vi "Word_Write_Text.vi"(8 "error in (no error)":errorcluster, 9 "text (\"\")":string, 10 "bookmark (\"\")":string="A_Faz_Frekans_3_3", 11 "report in":refnum<class "NI_report.lvclass">) -> (0 "error out":errorcluster, 3 "report out":refnum<class "NI_report.lvclass">)   [LabVIEW 2014]
doc: "This VI demonstrates the use of ActiveX to write a table into a Microsoft Excel worksheet."
uses:
  <vilib>/Utility/NIReport.llb/NI_report.lvclass
  <vilib>/Utility/NIReport.llb/Word/NI_Word.lvclass
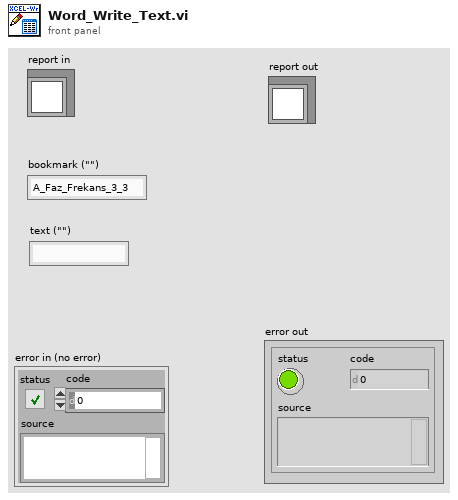
[diagram p1: front panel]
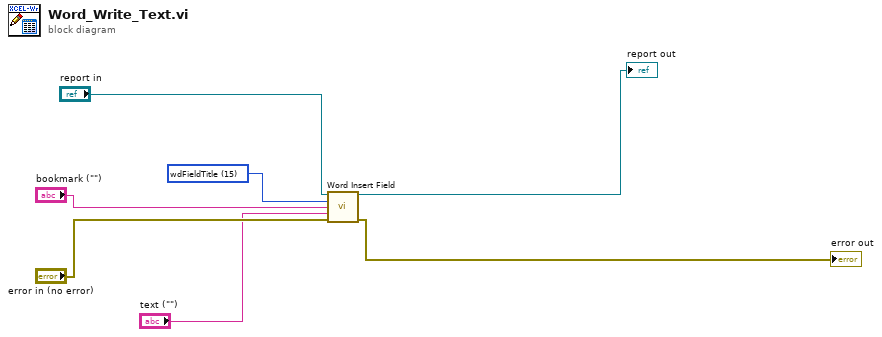
[diagram p0: block diagram]
diagram:
  w3 = 15 items=["wdFieldEmpty"=-1, "wdFieldRef"=3, "wdFieldIndexEntry"=4, "wdFieldFootnoteRef"=5, "wdFieldSet"=6, "wdFieldIf"=7, "wdFieldIndex"=8, "wdFieldTOCEntry"=9, "wdFieldStyleRef"=10, "wdFieldRefDoc"=11, "wdFieldSequence"=12, "wdFieldTOC"=13, "wdFieldInfo"=14, "wdFieldTitle"=15, "wdFieldSubject"=16, "wdFieldAuthor"=17, "wdFieldKeyWord"=18, "wdFieldComments"=19, "wdFieldLastSavedBy"=20, "wdFieldCreateDate"=21, "wdFieldSaveDate"=22, "wdFieldPrintDate"=23, "wdFieldRevisionNum"=24, "wdFieldEditTime"=25, "wdFieldNumPages"=26, "wdFieldNumWords"=27, "wdFieldNumChars"=28, "wdFieldFileName"=29, "wdFieldTemplate"=30, "wdFieldDate"=31, "wdFieldTime"=32, "wdFieldPage"=33, "wdFieldExpression"=34, "wdFieldQuote"=35, "wdFieldInclude"=36, "wdFieldPageRef"=37, "wdFieldAsk"=38, "wdFieldFillIn"=39, "wdFieldData"=40, "wdFieldNext"=41, "wdFieldNextIf"=42, "wdFieldSkipIf"=43, "wdFieldMergeRec"=44, "wdFieldDDE"=45, "wdFieldDDEAuto"=46, "wdFieldGlossary"=47, "wdFieldPrint"=48, "wdFieldFormula"=49, "wdFieldGoToButton"=50, "wdFieldMacroButton"=51, "wdFieldAutoNumOutline"=52, "wdFieldAutoNumLegal"=53, "wdFieldAutoNum"=54, "wdFieldImport"=55, "wdFieldLink"=56, "wdFieldSymbol"=57, "wdFieldEmbed"=58, "wdFieldMergeField"=59, "wdFieldUserName"=60, "wdFieldUserInitials"=61, "wdFieldUserAddress"=62, "wdFieldBarCode"=63, "wdFieldDocVariable"=64, "wdFieldSection"=65, "wdFieldSectionPages"=66, "wdFieldIncludePicture"=67, "wdFieldIncludeText"=68, "wdFieldFileSize"=69, "wdFieldFormTextInput"=70, "wdFieldFormCheckBox"=71, "wdFieldNoteRef"=72, "wdFieldTOA"=73, "wdFieldTOAEntry"=74, "wdFieldMergeSeq"=75, "wdFieldPrivate"=77, "wdFieldDatabase"=78, "wdFieldAutoText"=79, "wdFieldCompare"=80, "wdFieldAddin"=81, "wdFieldSubscriber"=82, "wdFieldFormDropDown"=83, "wdFieldAdvance"=84, "wdFieldDocProperty"=85, "wdFieldOCX"=87, "wdFieldHyperlink"=88, "wdFieldAutoTextList"=89, "wdFieldListNum"=90, "wdFieldHTMLActiveX"=91] ("type")
  n1 = call <vilib>:"Word Insert Field.vi"("report in"="report in", "type"=w3, "bookmark (\"\")"="bookmark (\"\")", "text (\"\")"="text (\"\")", "error in (no error)"="error in (no error)") -> ("report out"=→"report out":refnum<class "NI_report.lvclass">, "error out"=→"error out":errorcluster)  [unwired: 9 in]
